vi "Update States Data.vi"(8 "error in (no error)":errorcluster, 10 "State Map":map{string, string}(c390), 11 "List Seen Processes View Model In":refnum<class "Process Tree View Model.lvclass">) -> (0 "error out":errorcluster, 3 "List Seen Processes View Model Out":refnum<class "Process Tree View Model.lvclass">)   [LabVIEW 2020, in "Process Tree View Model.lvclass"]
uses:
  Process Tree View Model.lvclass
  Process Tree View Model.lvclass/Process Tree View Model.ctl
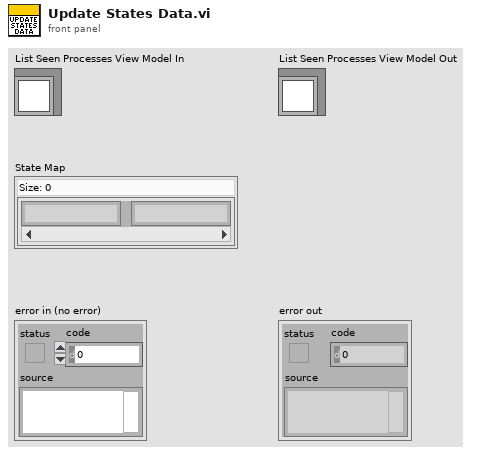
[diagram p1: front panel]
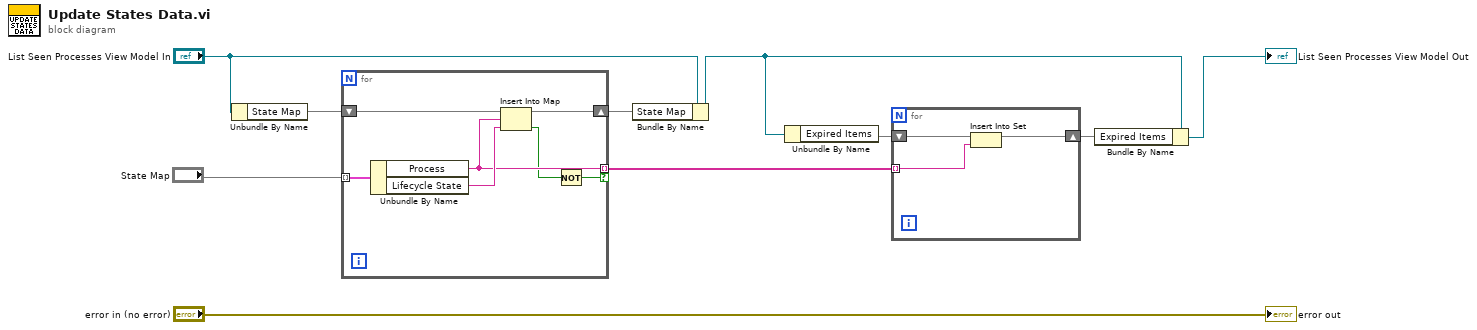
[diagram p0: block diagram]
diagram:
  n1 = Unbundle By Name("List Seen Processes View Model In") -> ("State Map"=w8:map{string, string})
  n2 = for {
    shift-right: [w14] -> w7
    shift-left: w8 -> [w16]
    tunnel: "State Map" -> [w17] mode=indexing
    tunnel: [w13] -> w1 mode=indexing if=w11
    n3 = Unbundle By Name(w17) -> ("Process"=w13:string, "Lifecycle State"=w15:string)
    n4 = Insert Into Map(map in=w16, key=w13, value=w15) -> (map out=w14:map{string, string}, value unchanged?=w12:bool)  [unwired: 1 out]
    n5 = Not(x=w12) -> (.not. x?=w11:bool)
  }
  n6 = Bundle By Name(cluster="List Seen Processes View Model In", "State Map"=w7) -> (w4:refnum<class "Process Tree View Model.lvclass">)
  n7 = Unbundle By Name(w4) -> ("Expired Items"=w5:set{string})
  n8 = for {
    shift-right: [w19] -> w2
    shift-left: w5 -> [w20]
    tunnel: w1 -> [w18] mode=indexing
    n9 = Insert Into Set(10:w18, 11:w20) -> (3:w19:set{string})  [unwired: 1 out]
  }
  n10 = Bundle By Name(cluster=w4, "Expired Items"=w2) -> (→"List Seen Processes View Model Out":refnum<class "Process Tree View Model.lvclass">)
  "error out" <- "error in (no error)"
